vi "Initialize.vi"(8 "error in (no error)":errorcluster, 11 "DAQ in":refnum<class "DAQ.lvclass">) -> (0 "error out":errorcluster, 3 "DAQ out":refnum<class "DAQ.lvclass">)   [LabVIEW 2020, in "DAQ.lvlib" / "DAQ.lvclass"]
uses:
  DAQ.lvclass
  Device/Device/Device.lvclass
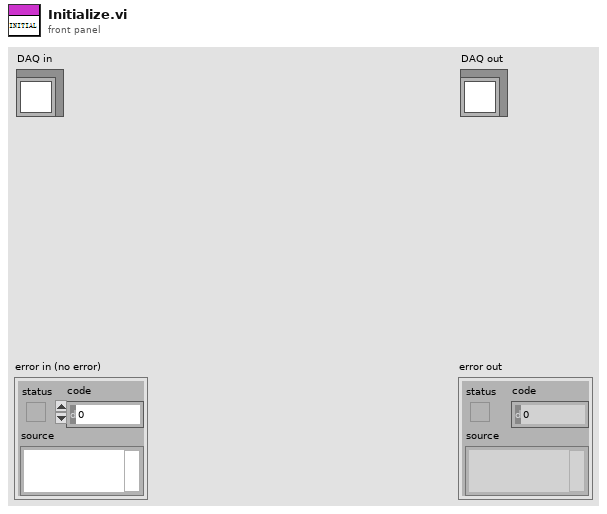
[diagram p1: front panel]
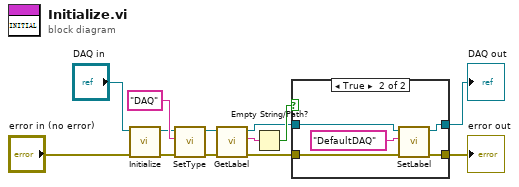
[diagram p0: block diagram]
diagram:
  n1 = call-parent "Initialize.vi"("error in (no error)"="error in (no error)", "GRMActor in"="DAQ in") -> ("error out"=w3:errorcluster, "GRMActor out"=w4:refnum<class "DAQ.lvclass">)  [unwired: 8 in]
  n2 = call-dynamic "SetType.vi"("error in (no error)"=w3, "Type"="DAQ", "GRMActor in"=w4) -> ("error out"=w11:errorcluster, "GRMActor out"=w9:refnum<class "DAQ.lvclass">)  [unwired: 7 in]
  n3 = call-dynamic "GetLabel.vi"("error in (no error)"=w11, "GRMActor in"=w9) -> ("error out"=w5:errorcluster, "Label"=w8:string, "GRMActor out"=w6:refnum<class "DAQ.lvclass">)  [unwired: 7 in]
  n4 = Empty String/Path?(string/path=w8) -> (empty?=w7:bool)
  n5 = case shown="True" w7 {
    tunnel: w6 -> [w15 w18]
    tunnel: w5 -> [w14 w20]
    tunnel: [w15 w17] -> w2
    tunnel: [w14 w19] -> w1
    frame False {
    }
    frame True {
      n6 = call-dynamic "SetLabel.vi"("error in (no error)"=w20, "Label"="DefaultDAQ", "GRMActor in"=w18) -> ("error out"=w19:errorcluster, "GRMActor out"=w17:refnum<class "DAQ.lvclass">)  [unwired: 7 in]
    }
  }
  "error out" <- w1
  "DAQ out" <- w2
